vi "niScope Direct DMA Multi Fetch Binary.vi"(0 "instrument handle":refnum<k15>, 1 "timeout":dbl=5.0 format="%.2f", 5 "channels":string="0", 9 "numSamples":i32=-1, 11 "error in":errorcluster, 12 "bufferSize":u32, 13 "bufferAddress":u32) -> (4 "instrument handle out":refnum<k15>, 6 "wfm info":T1(array[cluster]) {"reserved2" format="%.2f"; "reserved1" format="%.2f"; "offset" format="%^.3e"; "gain" format="%^.3e"; "xIncrement" format="%^.3e"; "relativeInitialX" format="%^.3e"; "absoluteInitialX" format="%^.3e"}, 10 "offset to first sample":i32[](array[numeric]), 15 "error out":errorcluster)   [LabVIEW 2013]
uses:
  niScope_32.dll
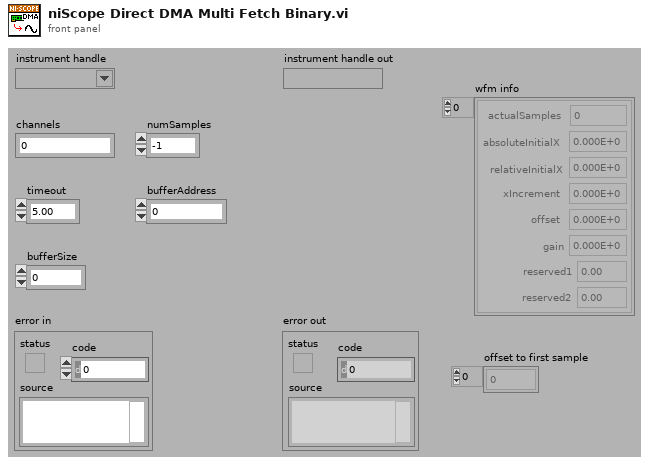
[diagram p1: front panel]
types:
  T1 = cluster{"actualSamples":i32, "absoluteInitialX":dbl, "relativeInitialX":dbl, "xIncrement":dbl, "offset":dbl, "gain":dbl, "reserved1":dbl, "reserved2":dbl}[]
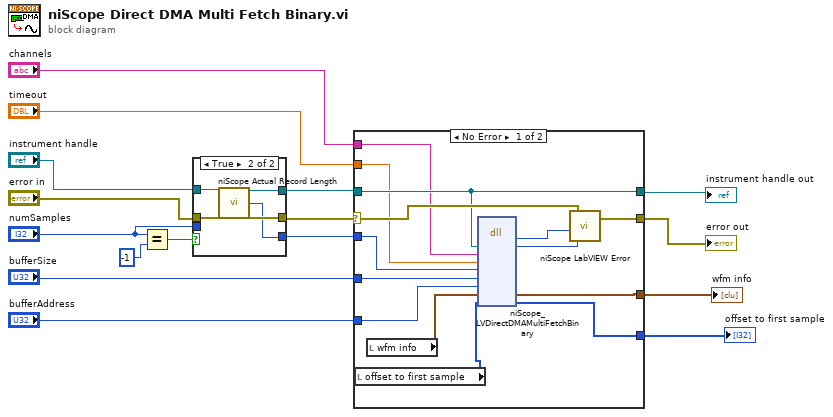
[diagram p0: block diagram]
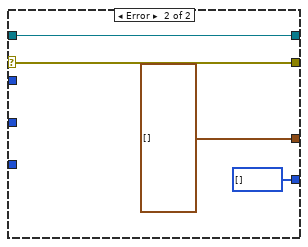
[diagram p3: hidden frame]
diagram:
  n1 = Equal?(x="numSamples", y=-1) -> (x = y?=w13:bool)
  n2 = case shown="True" w13 {
    tunnel: [w18 w24] -> w10
    tunnel: [w19 w23] -> w11
    tunnel: "numSamples" -> [w17 _]
    tunnel: [w17 w20] -> w9
    tunnel: "instrument handle" -> [w19 w22]
    tunnel: "error in" -> [w18 w21]
    frame False {
    }
    frame True {
      n3 = call <instrlib>:"niScope Actual Record Length.vi"("instrument handle"=w22, "error in"=w21) -> ("instrument handle out"=w23:refnum<k15>, "actual record length"=w20:i32, "error out"=w24:errorcluster)  [unwired: 11 in]
    }
  }
  n4 = case shown="No Error" w10 {
    selector: w10 -> [w35 w41]
    tunnel: [w36 w41] -> w16
    tunnel: w11 -> [w34 w42]
    tunnel: [w34 w42] -> w15
    tunnel: w9 -> [w31 _]
    tunnel: [w27 T1 [] ("wfm info")] -> w2
    tunnel: "timeout" -> [w33 _]
    tunnel: "channels" -> [w32 _]
    tunnel: "bufferSize" -> [w30 _]
    tunnel: [w29 u32[] [] ("offsetToFirstSample")] -> w1
    tunnel: "bufferAddress" -> [w28 _]
    frame No Error {
      n5 = local read "offset to first sample"() -> (w25:i32[])
      n6 = local read "wfm info"() -> (w26:T1)
      n7 = dll-call lib="niScope_*.*" fn="niScope_LVDirectDMAMultiFetchBinary"("instrument handle"=w34, "channel"=w32, "timeout"=w33, "numSamples"=w31, "bufferSize"=w30, "bufferAddress"=w28, "wfm_info"=w26, "offsetToFirstSample"=w25) -> ("status"=w38:i32, "instrument handle"=w37:u32, "wfm_info"=w27:T1, "offsetToFirstSample"=w29:i32[])  [unwired: 8 in, 2 out]
      n8 = call <instrlib>:"niScope LabVIEW Error.vi"("instrument handle"=w37, "niScope error code (0)"=w38, "error in (no error)"=w35) -> ("error out"=w36:errorcluster)  [unwired: 2 in]
    }
    frame Error {
    }
  }
  "instrument handle out" <- w15
  "error out" <- w16
  "wfm info" <- w2
  "offset to first sample" <- w1
